vi "SIM ChkTolerance.vi"(8 "Error In":errorcluster, 10 "relativeTolerance":dbl, 11 "absoluteTolerance":dbl) -> (0 "Error Out":errorcluster)   [LabVIEW 2014]
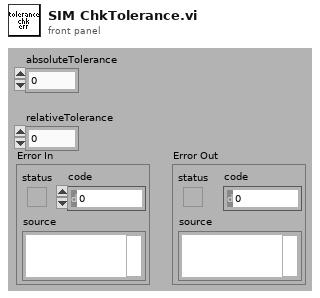
[diagram p1: front panel]
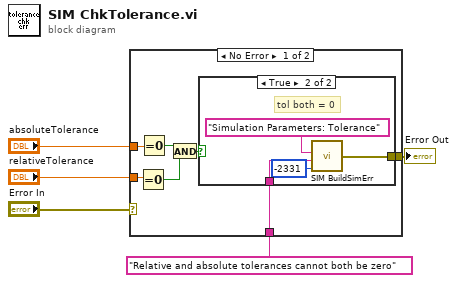
[diagram p0: block diagram]
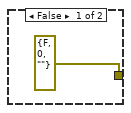
[diagram p2: hidden frame]
diagram:
  n1 = case shown="No Error" "Error In" {
    selector: "Error In" -> [_ w18]
    tunnel: [w12 w18] -> w5
    tunnel: "relativeTolerance" -> [w8 _]
    tunnel: "absoluteTolerance" -> [w7 _]
    tunnel: "Relative and absolute tolerances cannot both be zero" ("Additional Details") -> [w6 _]
    frame No Error {
      n2 = Equal To 0?(x=w8) -> (x = 0?=w9:bool)
      n3 = Equal To 0?(x=w7) -> (x = 0?=w10:bool)
      n4 = And(x=w10, y=w9) -> (x .and. y?=w11:bool)
      n5 = case shown="True" w11 {
        tunnel: [errorcluster {"status"=FALSE, "code"=0, "source"=""} ("Error Cluster") w17] -> w12
        tunnel: w6 -> [_ w15]
        frame False {
        }
        frame True {
          # "tol both = 0"
          n6 = call "SIM BuildSimErr.vi"("error.code"=-2331, "Additional Details"=w15, "Block Name"="Simulation Parameters: Tolerance" ("CallChain")) -> ("Error Cluster"=w17:errorcluster)  [unwired: 1 in]
        }
      }
    }
    frame Error {
    }
  }
  "Error Out" <- w5
